vi "IR RawData Event Example.vi"() -> ()   [LabVIEW 2012, in "Phidget IR.lvlib"]
uses:
  <instrlib>/Phidgets/Phidget IR/Phidget IR.lvlib
  <instrlib>/Phidgets/Phidget IR/Public/IRStart.vi
  <instrlib>/Phidgets/Phidget IR/Public/IRClose.vi
  <instrlib>/Phidgets/Phidget Common/Phidget Common.lvlib
panel:
  in  "Device Info":T1={"Serial Number"=-1, "Channel"=0, "Port"=0}
  out "RawData":string
  out "RawData":u32[](array[numeric])
  out "Event?":bool
  in  "stop":bool
  out "Serial Number Return":i32
  out "error out":errorcluster
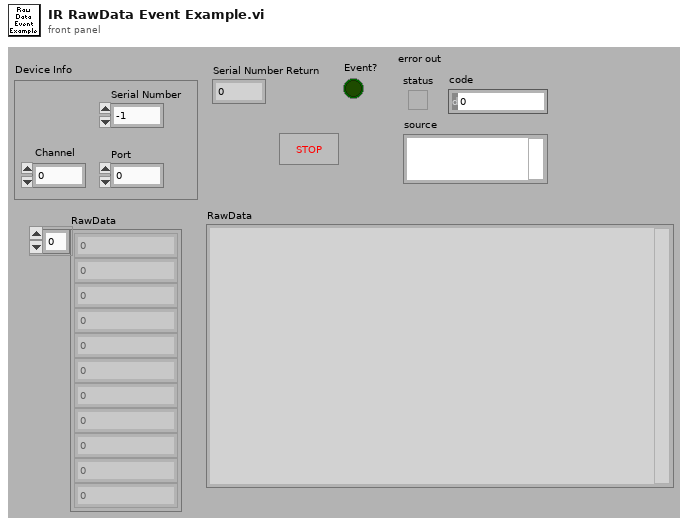
[diagram p1: front panel]
types:
  T1 = cluster{"Serial Number":i32, "Channel":i32, "Port":i32}
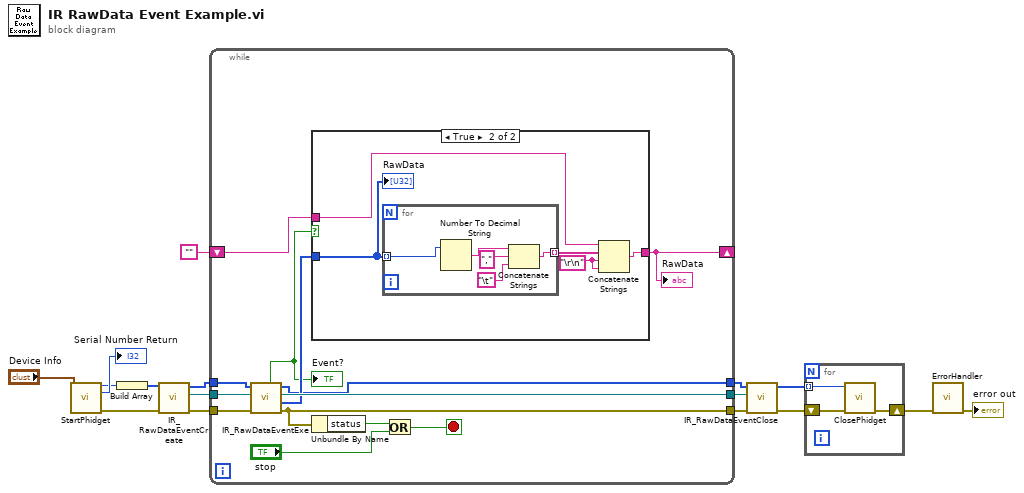
[diagram p0: block diagram]
diagram:
  n1 = call-poly <instrlib>:"StartPhidget.vi"("Device Info"="Device Info") -> ("Phidget ID"=w5:u64, "Serial Number Return"=→"Serial Number Return":i32, "error out"=w14:errorcluster)  [unwired: 11 in, 1 out]
  n2 = Build Array(w5) -> (w4:u64[])
  n3 = call <instrlib>:"IR_RawDataEventCreate.vi"("error in (no error)"=w14, "Devices In"=w4) -> ("error out"=w13:errorcluster, "Event Registration Refnum"=w12:refnum<event-registration>, "Devices Out"=w11:u64[])  [unwired: 7 in]
  n4 = while {
    tunnel: w11 -> [w22]
    tunnel: w13 -> [w28]
    tunnel: w12 -> [w29]
    tunnel: [w27] -> w8
    tunnel: [w26] -> w10
    tunnel: [w17] -> w6
    shift-right: [w18] -> _
    shift-left: "" -> [w20]
    stop <- w23 stop-if-true
    n5 = call <instrlib>:"IR_RawDataEventExe.vi"("error in (no error)"=w28, "Event Registration Refnum In"=w29, "Devices In"=w22) -> ("error out"=w26:errorcluster, "Raw Data"=w21:u32[], "Event Registration Refnum Out"=w27:refnum<event-registration>, "Devices Out"=w17:u64[], "Event?"=w19:bool)  [unwired: 2 in, 2 out]
    "Event?" <- w19
    n6 = case shown="True" w19 {
      tunnel: w21 -> [_ w33]
      tunnel: w20 -> [w30 w35]
      tunnel: [w30 w34] -> w18
      frame False {
      }
      frame True {
        w31 = "\r\n"
        n7 = for {
          tunnel: w33 -> [w40] mode=indexing
          tunnel: [w37] -> w32 mode=indexing
          n8 = Number To Decimal String(number=w40) -> (decimal integer string=w38:string)  [unwired: 1 in]
          n9 = Concatenate Strings(w38, "," ("string"), "\t") -> (w37:string)
        }
        n10 = Concatenate Strings(w35, w32, w31, w31) -> (w34:string)
        "RawData" <- w33
      }
    }
    "RawData" <- w18
    n11 = Unbundle By Name(w26) -> ("status"=w25:bool)
    n12 = Or(x=w25, y="stop") -> (x .or. y?=w23:bool)
  }
  n13 = call <instrlib>:"IR_RawDataEventClose.vi"("error in (no error)"=w10, "Event Registration Refnum In"=w8, "Devices In"=w6) -> ("error out"=w1:errorcluster, "Devices Out"=w9:u64[])  [unwired: 7 in]
  n14 = for {
    tunnel: w9 -> [w42] mode=indexing
    shift-right: [w43] -> w2
    shift-left: w1 -> [w41]
    n15 = call-poly <instrlib>:"ClosePhidget.vi"("error in"=w41, "Device In"=w42) -> ("error out"=w43:errorcluster)  [unwired: 9 in]
  }
  n16 = call <instrlib>:"ErrorHandler.vi"("error in"=w2) -> ("error out"=→"error out":errorcluster)  [unwired: 9 in, 1 out]
